vi "Storage ReadData.vi"() -> (0 "Image Data":dbl[][](array[numeric]), 1 "cancelled":bool, 2 "Data type ID":string, 3 "Acoustic Data":T2, 4 "path":path, 5 "Data Referenzen":T1)   [LabVIEW 2022 SP3]
uses:
  Data Record.ctl
  RF Data Value Reference.ctl
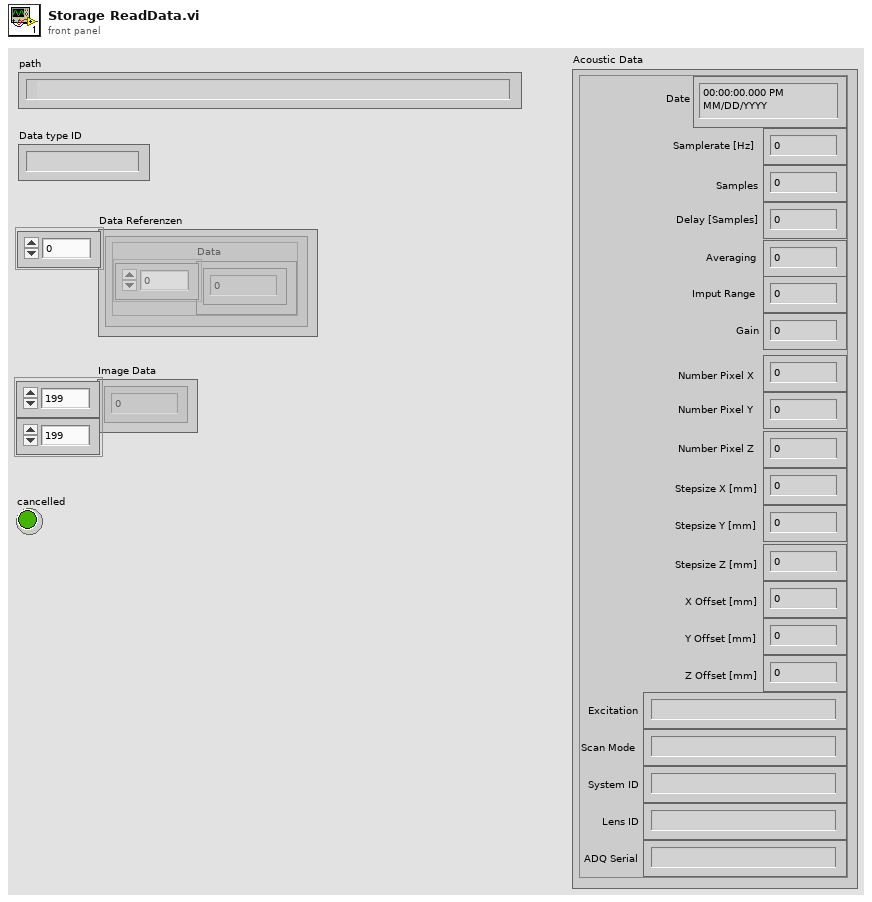
[diagram p1: front panel]
types:
  T1 = typedef "RF Data Value Reference.ctl" = cluster{"Data":sgl[]}[]
  T2 = typedef "Data Record.ctl" = cluster{"Samplerate [Hz] ":dbl, "Delay [Samples]":i32, "Stepsize X [mm]":dbl, "Stepsize Y [mm]":dbl, "Z Offset [mm]":dbl, "Number Pixel X":i32, "Samples":i32, "Number Pixel Y":i32, "System ID":string, "Lens ID":string, "Date":timestamp, "X Offset [mm]":dbl, "Y Offset [mm]":dbl, "Scan Mode":string, "Excitation":string, "Gain":dbl, "Imput Range":dbl, "Averaging":i32, "ADQ Serial":string, "Stepsize Z [mm]":dbl, "Number Pixel Z":i32}
  T3 = enum16{"big-endian, network order", "native, host order", "little-endian"}
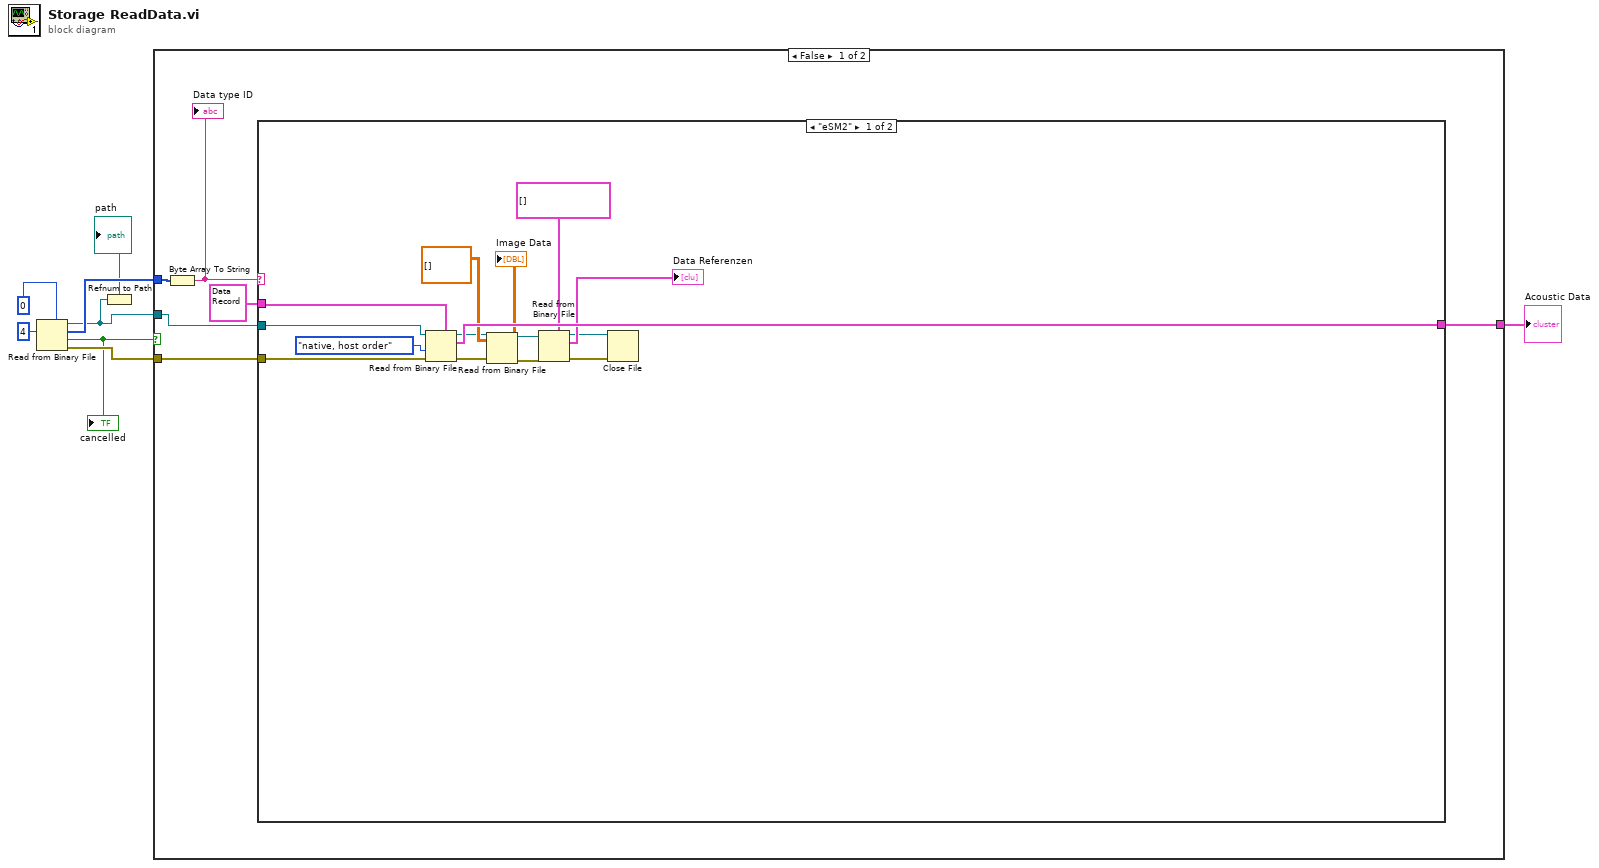
[diagram p0: block diagram]
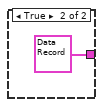
[diagram p3: hidden frame]
diagram:
  n1 = Read from Binary File(5:u8 0, 10:4 ("count (1)")) -> (0:w5:errorcluster, 1:w3:bool, 2:w6:u8[], 3:w2:refnum<file>)  [unwired: 4 in]
  "cancelled" <- w3
  n2 = Refnum to Path(1:w2) -> (0:→"path":path)
  n3 = case shown="False" w3 {
    tunnel: w2 -> [w14 _]
    tunnel: w6 -> [w13 _]
    tunnel: w5 -> [w11 _]
    tunnel: [w10 T2 {"Samplerate [Hz] "=0.0, "Delay [Samples]"=0, "Stepsize X [mm]"=0.0, "Stepsize Y [mm]"=0.0, "Z Offset [mm]"=0.0, "Number Pixel X"=0, "Samples"=0, "Number Pixel Y"=0, "System ID"="", "Lens ID"="", "Date"=timestamp(0 s since 1904-01-01), "X Offset [mm]"=0.0, "Y Offset [mm]"=0.0, "Scan Mode"="", "Excitation"="", "Gain"=0.0, "Imput Range"=0.0, "Averaging"=0, "ADQ Serial"="", "Stepsize Z [mm]"=0.0, "Number Pixel Z"=0} ("Acoustic Data")] -> w4
    frame False {
      n4 = Byte Array To String(unsigned byte array=w13) -> (string=w12:string)
      "Data type ID" <- w12
      n5 = case shown="\"eSM2\"" w12 {
        tunnel: w14 -> [w28 _]
        tunnel: w11 -> [w29 _]
        tunnel: T2 {"Samplerate [Hz] "=0.0, "Delay [Samples]"=0, "Stepsize X [mm]"=0.0, "Stepsize Y [mm]"=0.0, "Z Offset [mm]"=0.0, "Number Pixel X"=0, "Samples"=0, "Number Pixel Y"=0, "System ID"="", "Lens ID"="", "Date"=timestamp(0 s since 1904-01-01), "X Offset [mm]"=0.0, "Y Offset [mm]"=0.0, "Scan Mode"="", "Excitation"="", "Gain"=0.0, "Imput Range"=0.0, "Averaging"=0, "ADQ Serial"="", "Stepsize Z [mm]"=0.0, "Number Pixel Z"=0} ("Acoustic Data") -> [w26 w30]
        tunnel: [w25 w30] -> w10
        frame "eSM2" {
          n6 = Read from Binary File(5:w26, 8:w29, 9:T3."native, host order" ("byte order (0:big-endian, network order)"), 11:w28) -> (0:w20:errorcluster, 2:w25:T2, 3:w16:refnum<file>)  [unwired: 2 in, 1 out]
          n7 = Read from Binary File(5:dbl[][] [], 8:w20, 11:w16) -> (0:w19:errorcluster, 2:→"Image Data":dbl[][], 3:w15:refnum<file>)  [unwired: 3 in, 1 out]
          n8 = Read from Binary File(5:T1 [] ("Data Referenzen"), 8:w19, 11:w15) -> (0:w21:errorcluster, 2:→"Data Referenzen":T1, 3:w22:refnum<file>)  [unwired: 3 in, 1 out]
          n9 = Close File(refnum=w22, error in=w21) -> ()  [unwired: 2 out]
        }
        frame "AAA", Default {
        }
      }
    }
    frame True {
    }
  }
  "Acoustic Data" <- w4
